vi "Page_Destination_Update_Display.vi"(8 "error in (no error)":errorcluster, 9 "ctlReferences":T1, 11 "AB_Dest_App in":refnum<class "AB_Dest_LegacyApp.lvclass">) -> (0 "error out":errorcluster, 3 "AB_Dest_App out":refnum<class "AB_Dest_LegacyApp.lvclass">)   [LabVIEW 2020, in "AB_Dest_LegacyApp.lvclass"]
uses:
  <vilib>/AppBuilder/AB_Classes/Destination/Dest_LegacyApplication/AB_Dest_LegacyApp.lvclass
  <resource>/Framework/Providers/Builds/AppBuilder/AB_UI_Page_Destination_References.ctl
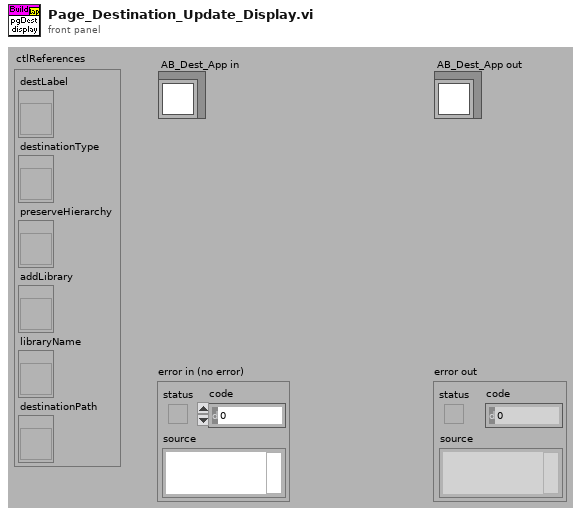
[diagram p1: front panel]
types:
  T1 = typedef "AB_UI_Page_Destination_References.ctl" = cluster{"destLabel":refnum<vi>, "destinationType":refnum<vi>, "preserveHierarchy":refnum<vi>, "addLibrary":refnum<vi>, "libraryName":refnum<vi>, "destinationPath":refnum<vi>}
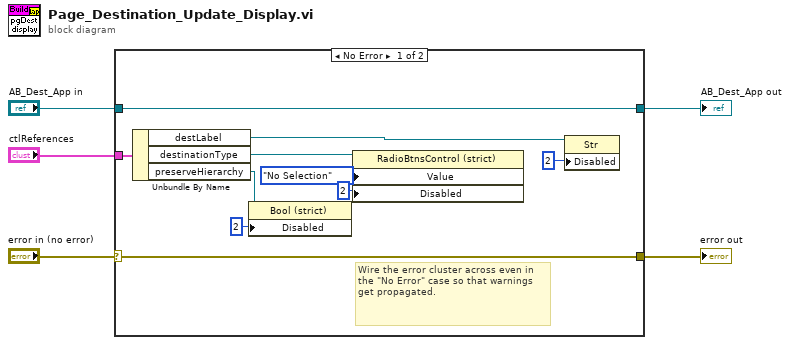
[diagram p0: block diagram]
diagram:
  n1 = case shown="No Error" "error in (no error)" {
    selector: "error in (no error)" -> [w14 w17]
    tunnel: [w14 w17] -> w3
    tunnel: [w15 w16] -> w4
    tunnel: "AB_Dest_App in" -> [w15 w16]
    tunnel: "ctlReferences" -> [w11 _]
    frame No Error {
      # "Wire the error cluster across even in the \"No Error\" case so that warnings get propagated."
      n2 = Unbundle By Name(w11) -> ("destLabel"=w9:refnum<vi>, "destinationType"=w10:refnum<vi>, "preserveHierarchy"=w7:refnum<vi>)
      n3 = property class="Bool (strict)"(reference=w7, "Disabled"=u8 2) -> ()  [unwired: 1 in, 2 out]
      n4 = property class="RadioBtnsControl (strict)"(reference=w10, "Value"=enum32{"No Selection", "Directory", "LLB"}."No Selection", "Disabled"=u8 2) -> ()  [unwired: 1 in, 2 out]
      n5 = property class="Str"(reference=w9, "Disabled"=u8 2) -> ()  [unwired: 1 in, 2 out]
    }
    frame Error {
    }
  }
  "error out" <- w3
  "AB_Dest_App out" <- w4
